vi "Write Message Enqueuer.vi"(8 "error in (no error)":errorcluster, 10 "Actor Framework:Message Enqueuer":refnum<class "Message Enqueuer.lvclass">, 11 "Iteration Msg in":refnum<class "Abstract Iteration Msg.lvclass">) -> (0 "error out":errorcluster, 3 "Iteration Msg out":refnum<class "Abstract Iteration Msg.lvclass">)   [LabVIEW 2023, in "Iterator Actor.lvlib" / "Abstract Iteration Msg.lvclass"]
uses:
  Abstract Iteration Msg.lvclass
  <vilib>/ActorFramework/Message Enqueuer/Message Enqueuer.lvclass
  Abstract Iteration Msg.lvclass/Abstract Iteration Msg.ctl
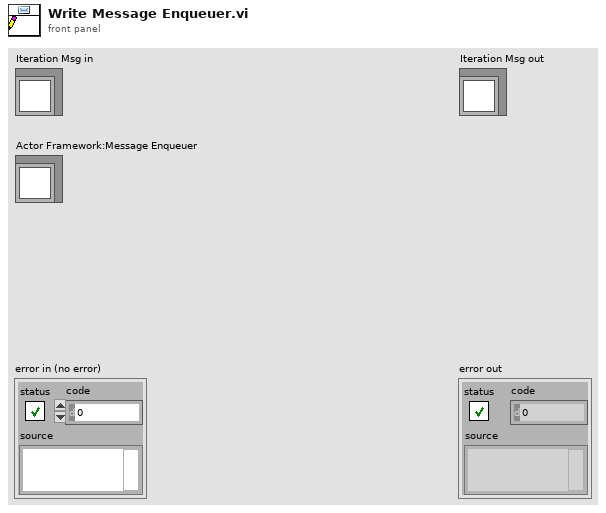
[diagram p1: front panel]
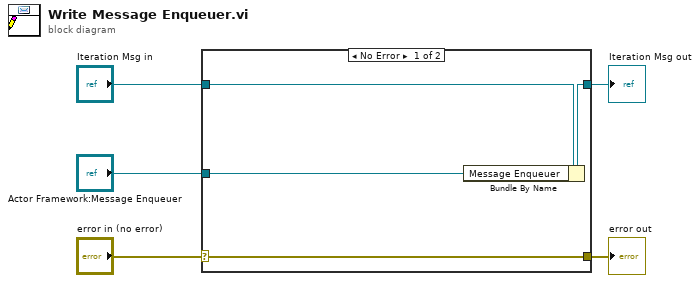
[diagram p0: block diagram]
diagram:
  n1 = case shown="No Error" "error in (no error)" {
    selector: "error in (no error)" -> [w9 w10]
    tunnel: [w9 w10] -> w4
    tunnel: [w7 w11] -> w2
    tunnel: "Iteration Msg in" -> [w8 w11]
    tunnel: "Actor Framework:Message Enqueuer" -> [w6 _]
    frame No Error {
      n2 = Bundle By Name(cluster=w8, "Message Enqueuer"=w6) -> (w7:refnum<class "Abstract Iteration Msg.lvclass">)
    }
    frame Error {
    }
  }
  "error out" <- w4
  "Iteration Msg out" <- w2
